vi "numCmd_Send_OneDbl.vi"(7 "Command Name":string, 11 "Value":dbl) -> (0 "error out":errorcluster)   [LabVIEW 2019, in "Trajectory_Library.lvlib"]
uses:
  Trajectory_Library.lvlib
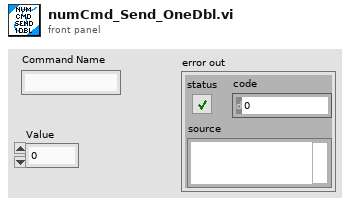
[diagram p1: front panel]
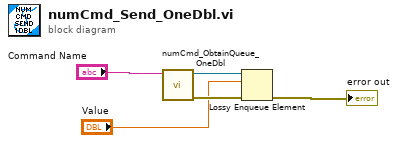
[diagram p0: block diagram]
diagram:
  n1 = call "numCmd_ObtainQueue_OneDbl.vi"("Command Name"="Command Name") -> ("error out"=w4:errorcluster, "queue out"=w5:refnum<queue>)  [unwired: 9 in]
  n2 = Lossy Enqueue Element(queue=w5, element="Value", error in (no error)=w4) -> (error out=→"error out":errorcluster)  [unwired: 3 out]
